vi "GFITS_LibMoveHdu.vi"(8 "error in (no error)":errorcluster, 9 "hdutype":i32, 10 "hdunum":i32, 11 "ref":u64) -> (0 "error out":errorcluster, 2 "return value":i32, 3 "ref out":u64)   [LabVIEW 2016]
uses:
  c/lib/libgfits.so
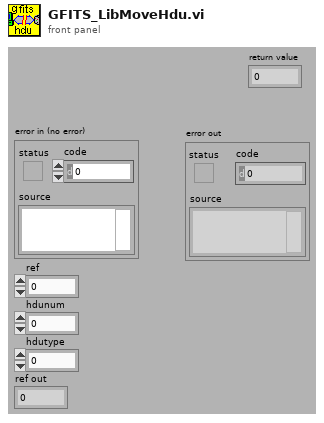
[diagram p1: front panel]
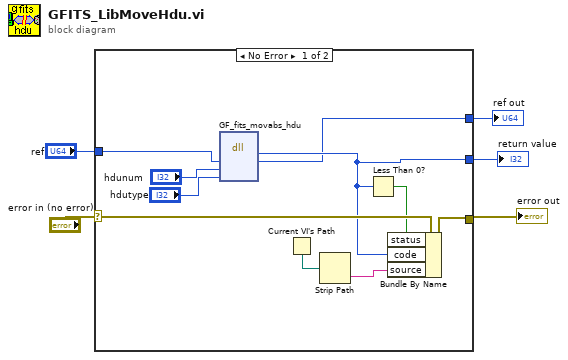
[diagram p0: block diagram]
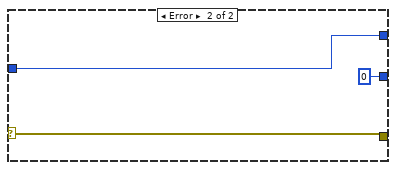
[diagram p2: hidden frame]
diagram:
  n1 = case shown="No Error" "error in (no error)" {
    selector: "error in (no error)" -> [w15 w18]
    tunnel: [w8 0] -> w5
    tunnel: [w11 w18] -> w3
    tunnel: [w7 w16] -> w2
    tunnel: "ref" -> [w6 w16]
    frame No Error {
      n2 = dll-call lib="home/simager/panview/PAN/Modules/GFITS/private/c/lib/libgfits.so" fn="GF_fits_movabs_hdu"("ref"=w6, "hdunum"="hdunum", "hdutype"="hdutype") -> ("return type"=w8:i32, "ref"=w7:u64)  [unwired: 5 in, 2 out]
      n3 = Current VI's Path() -> (path=w13:path)
      n4 = Strip Path(path=w13) -> (name=w12:string)  [unwired: 1 out]
      n5 = Less Than 0?(x=w8) -> (x < 0?=w14:bool)
      n6 = Bundle By Name(cluster=w15, "status"=w14, "code"=w8, "source"=w12) -> (w11:errorcluster)
    }
    frame Error {
    }
  }
  "return value" <- w5
  "error out" <- w3
  "ref out" <- w2
